vi "ProtectSources.vi"(1 "数字输入保护信号":bool[](array[boolean]), 2 "模拟输入保护信号":dbl[](array[numeric]), 3 "模拟保护信号设定值":cluster{"设定值":dbl, "保护配置规则":bool}) -> (0 "故障状态指示":cluster{"模拟信号故障？":bool, "数字信号故障？":bool})   [LabVIEW 2018]
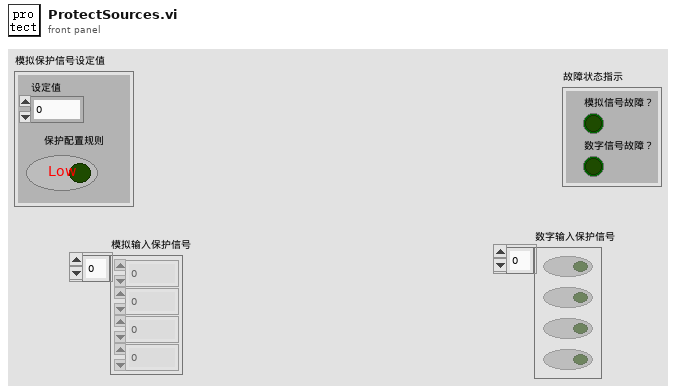
[diagram p1: front panel]
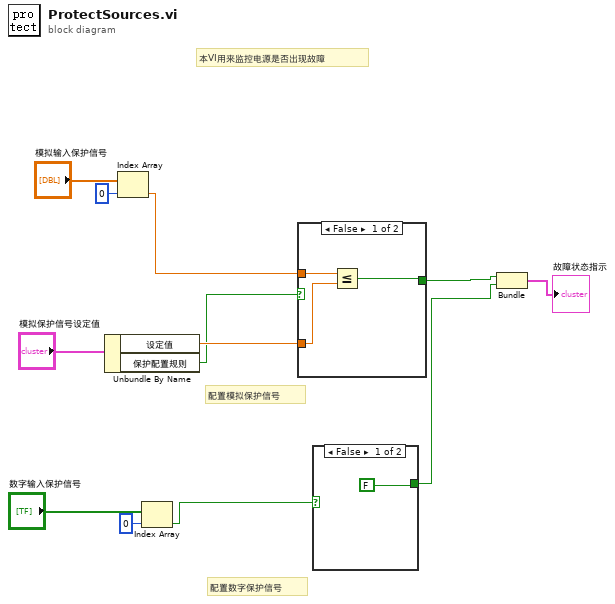
[diagram p0: block diagram]
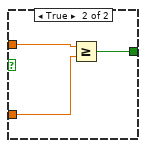
[diagram p2: hidden frame]
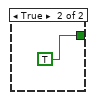
[diagram p3: hidden frame]
diagram:
  # "配置数字保护信号"
  # "配置模拟保护信号"
  # "本VI用来监控电源是否出现故障"
  n1 = Unbundle By Name("模拟保护信号设定值") -> ("设定值"=w11:dbl, "保护配置规则"=w1:bool)
  n2 = Index Array(array="模拟输入保护信号", index=0) -> (element=w5:dbl)
  n3 = Index Array(array="数字输入保护信号", index=0) -> (element=w2:bool)
  n4 = case shown="False" w1 {
    tunnel: w11 -> [w15 w18]
    tunnel: [w14 w17] -> w10
    tunnel: w5 -> [w13 w16]
    frame False {
      n5 = Less Or Equal?(x=w13, y=w15) -> (x <= y?=w14:bool)
    }
    frame True {
      n6 = Greater Or Equal?(x=w16, y=w18) -> (x >= y?=w17:bool)
    }
  }
  n7 = case shown="False" w2 {
    tunnel: [FALSE TRUE] -> w9
    frame False {
    }
    frame True {
    }
  }
  n8 = Bundle(w10, w9) -> (→"故障状态指示":cluster{bool, bool})  [unwired: 1 in]
